vi "SVX Convert Waterfall to Colormap.vi"(7 "plot type":T1(ring), 8 "error in (no error)":errorcluster, 11 "waterfall graph data":T3) -> (0 "error out":errorcluster, 1 "y-axis unit label":string, 2 "x-axis unit label":string, 3 "colormap":T2, 4 "z-axis unit label":string)   [LabVIEW 2017, in "SoundVib_SpectralDisplay.lvlib"]
doc: "Converts Waterfall Graph data to Colormap data."
uses:
  <vilib>/addons/Sound and Vibration/Order Analysis/Data Presentation/SoundVib_SpectralDisplay.lvlib
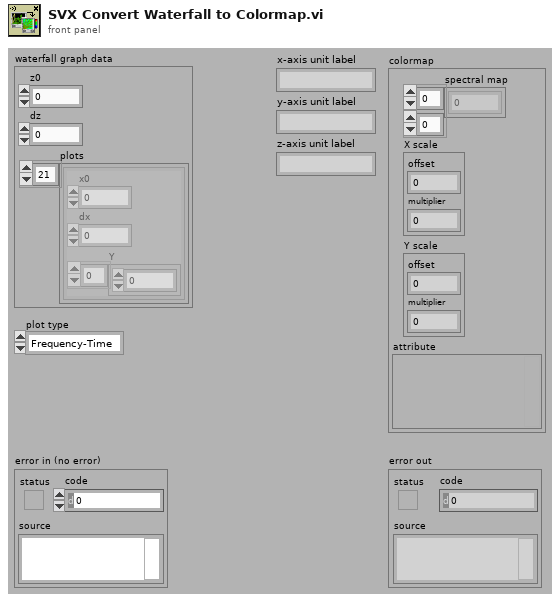
[diagram p1: front panel]
types:
  T1 = enum16{"Frequency-Time", "Time-Frequency", "Order-Time", "Time-Order", "Frequency-RPM", "RPM-Frequency", "Order-RPM", "RPM-Order"}
  T2 = cluster{"spectral map":dbl[][], "X scale":cluster{"offset":dbl, "multiplier":dbl}, "Y scale":cluster{"offset":dbl, "multiplier":dbl}, "attribute":variant}
  T3 = cluster{"z0":dbl, "dz":dbl, "plots":cluster{"x0":dbl, "dx":dbl, "Y":dbl[]}[]}
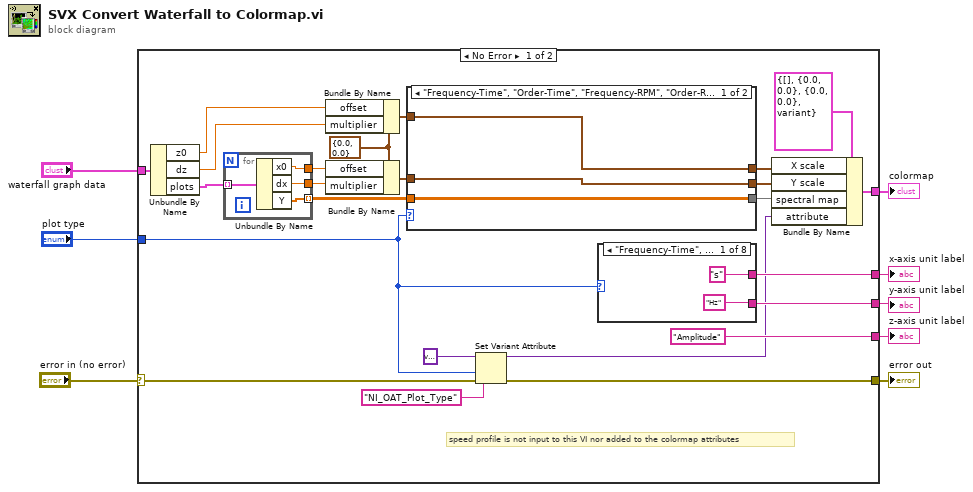
[diagram p0: block diagram]
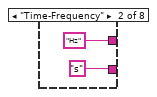
[diagram p2: hidden frame]
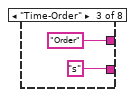
[diagram p3: hidden frame]
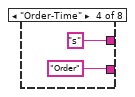
[diagram p4: hidden frame]
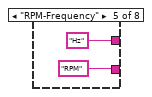
[diagram p5: hidden frame]
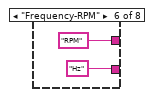
[diagram p6: hidden frame]
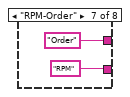
[diagram p7: hidden frame]
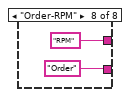
[diagram p8: hidden frame]
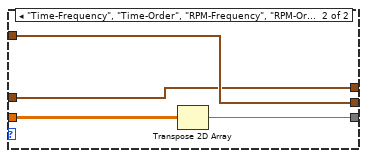
[diagram p9: hidden frame]
diagram:
  n1 = case shown="No Error" "error in (no error)" {
    selector: "error in (no error)" -> [w10 w60]
    tunnel: "waterfall graph data" -> [w31 _]
    tunnel: [w9 w60] -> w7
    tunnel: [w17 _] -> w6
    tunnel: "plot type" -> [w16 _]
    tunnel: [w15 _] -> w4
    tunnel: [w14 _] -> w3
    tunnel: ["Amplitude" ("Z axis unit label") _] -> w2
    frame No Error {
      w26 = cluster{"offset":dbl, "multiplier":dbl} {"offset"=0.0, "multiplier"=0.0} ("X scale")
      # "speed profile is not input to this VI nor added to the colormap attributes"
      n2 = Unbundle By Name(w31) -> ("z0"=w12:dbl, "dz"=w25:dbl, "plots"=w29:cluster{"x0":dbl, "dx":dbl, "Y":dbl[]}[])
      n3 = for {
        tunnel: w29 -> [w52] mode=indexing
        tunnel: [w51] -> w28 mode=indexing
        tunnel: [w50] -> w23
        tunnel: [w49] -> w24
        n4 = Unbundle By Name(w52) -> ("x0"=w50:dbl, "dx"=w49:dbl, "Y"=w51:dbl[])
      }
      n5 = Bundle By Name(cluster=w26, "offset"=w12, "multiplier"=w25) -> (w21:cluster{"offset":dbl, "multiplier":dbl})
      n6 = Bundle By Name(cluster=w26, "offset"=w23, "multiplier"=w24) -> (w22:cluster{"offset":dbl, "multiplier":dbl})
      n7 = case shown="\"Frequency-Time\", \"Order-Time\", \"Frequency-RPM\", \"Order-RPM\", Default" w16 {
        tunnel: w28 -> [w53 w59]
        tunnel: [w53 w58] -> w20
        tunnel: w21 -> [w55 w57]
        tunnel: [w54 w57] -> w18
        tunnel: w22 -> [w54 w56]
        tunnel: [w55 w56] -> w19
        frame "Frequency-Time", "Order-Time", "Frequency-RPM", "Order-RPM", Default {
        }
        frame "Time-Frequency", "Time-Order", "RPM-Frequency", "RPM-Order" {
          n8 = Transpose 2D Array(2D array=w59) -> (transposed array=w58:dbl[][])
        }
      }
      n9 = Set Variant Attribute(Variant=variant ("variant"), name="NI_OAT_Plot_Type", value=w16, error in=w10) -> (Variant out=w11:variant, error out=w9:errorcluster)  [unwired: 1 out]
      n10 = case shown="\"Frequency-Time\", Default" w16 {
        tunnel: ["s" ("name") "Hz" ("name") "Order" ("name") "s" ("name") "Hz" ("name") "RPM" ("name") "Order" ("name") "RPM" ("name")] -> w15
        tunnel: ["Hz" ("name") "s" ("name") "s" ("name") "Order" ("name") "RPM" ("name") "Hz" ("name") "RPM" ("name") "Order" ("name")] -> w14
        frame "Frequency-Time", Default {
        }
        frame "Time-Frequency" {
        }
        frame "Time-Order" {
        }
        frame "Order-Time" {
        }
        frame "RPM-Frequency" {
        }
        frame "Frequency-RPM" {
        }
        frame "RPM-Order" {
        }
        frame "Order-RPM" {
        }
      }
      n11 = Bundle By Name(cluster=T2 {"spectral map"=[], "X scale"={"offset"=0.0, "multiplier"=0.0}, "Y scale"={"offset"=0.0, "multiplier"=0.0}, "attribute"=variant} ("Colormap 2"), "X scale"=w19, "Y scale"=w18, "spectral map"=w20, "attribute"=w11) -> (w17:T2)
    }
    frame Error {
    }
  }
  "colormap" <- w6
  "error out" <- w7
  "x-axis unit label" <- w4
  "y-axis unit label" <- w3
  "z-axis unit label" <- w2
